vi "Keith 7001 Send Trigger.vi"(0 "GPIB address":string="7", 2 "error in":T1) -> (1 "error out":T1)   [LabVIEW 2019]
doc: "This VI for the Keithley 7001 Switch System sends a trigger to the device."
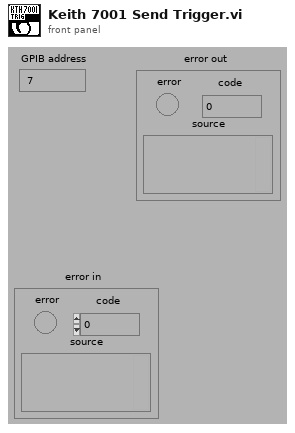
[diagram p1: front panel]
types:
  T1 = cluster{"error":bool, "code":i32, "source":string}
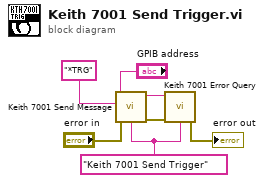
[diagram p0: block diagram]
diagram:
  w2 = "Keith 7001 Send Trigger"
  n1 = call "Keith 7001 Send Message.vi"("address string"="GPIB address", "write buffer"="*TRG", "source"=w2, "error in"="error in") -> ("address out"=w3:string, "error out"=w4:T1)  [unwired: 2 in, 2 out]
  n2 = call "Keith 7001 Error Query.vi"("GPIB address"=w3, "error in"=w4, "source"=w2) -> ("error out"=→"error out":T1)  [unwired: 2 out]
